vi "SingleStationGasMeter_NonNIHW.vi"() -> ()   [LabVIEW 2012]
uses:
  <vilib>/ULx/Create Channel.llb/ULx Create Channel (AI-Voltage-Basic).vi
  <vilib>/ULx/Read.llb/ULx Read (Analog DBL 1Chan 1Samp).vi
panel:
  out "ANSI Placeholder 3":dbl
  out "Start Time ANSI 3":dbl
  out "ANSI Placeholder 2":dbl
  out "Start Time ANSI 2":dbl
  out "Meter 2 Present":bool
  out "Meter 1 Present":bool
  out "Meter Type 2":string
  out "Meter Type 1":string
  out "Meter 2 Size":dbl
  out "Meter 1 Size":dbl
  out "ANSI Placeholder":dbl
  out "Start Time ANSI":dbl
  in  "Start ANSI":bool
  out "ANSI Average (BTU/hr)":dbl format="%#_5g"
  out "30 Second Average (BTU/hr)":dbl format="%#_5g"
  out "15 Second Average (BTU/hr)":dbl format="%#_5g"
  out "Reference6":dbl
  out "Reference5":dbl
  out "Reference4":dbl
  out "Reference3":dbl
  out "Reference2":dbl
  out "Reference1":dbl
  out "Time":dbl
  out "Num Record":dbl
  in  "HeatingValueLP":dbl=2450.0 min=2400.0 max=2600.0 step=5.0
  out "Output 6":dbl min=0.0 max=5.0 step=0.01
  out "Output 5":dbl min=0.0 max=5.0 step=0.01
  out "Output 4":dbl min=0.0 max=5.0 step=0.01
  out "Output 3":dbl min=0.0 max=5.0 step=0.01
  out "Output 2":dbl min=0.0 max=5.0 step=0.01
  out "Output 1":dbl min=0.0 max=5.0 step=0.01
  out "Signal":bool
  in  "Record":bool
  out "File Path":path
  out "CF/HR":dbl format="%#_2g"
  out "HV":dbl
  in  "HeatingValueNG":dbl=990.0 min=990.0 max=1150.0 step=1.0
  out "Meter ID":dbl
  out "Gas":string
  out "DisplayChart":cluster{"Flow Rate":dbl}(graph)
  out "Flow Rate":dbl format="%#_5g"
  # "Heating Value"
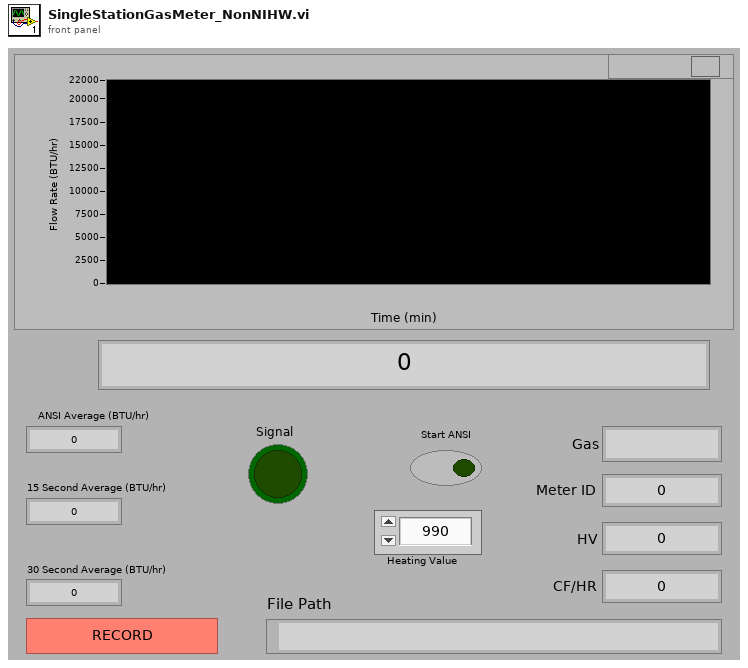
[diagram p1: front panel]
types:
  T1 = enum16{"open", "replace", "create", "open or create", "replace or create", "replace or create with confirmation"}
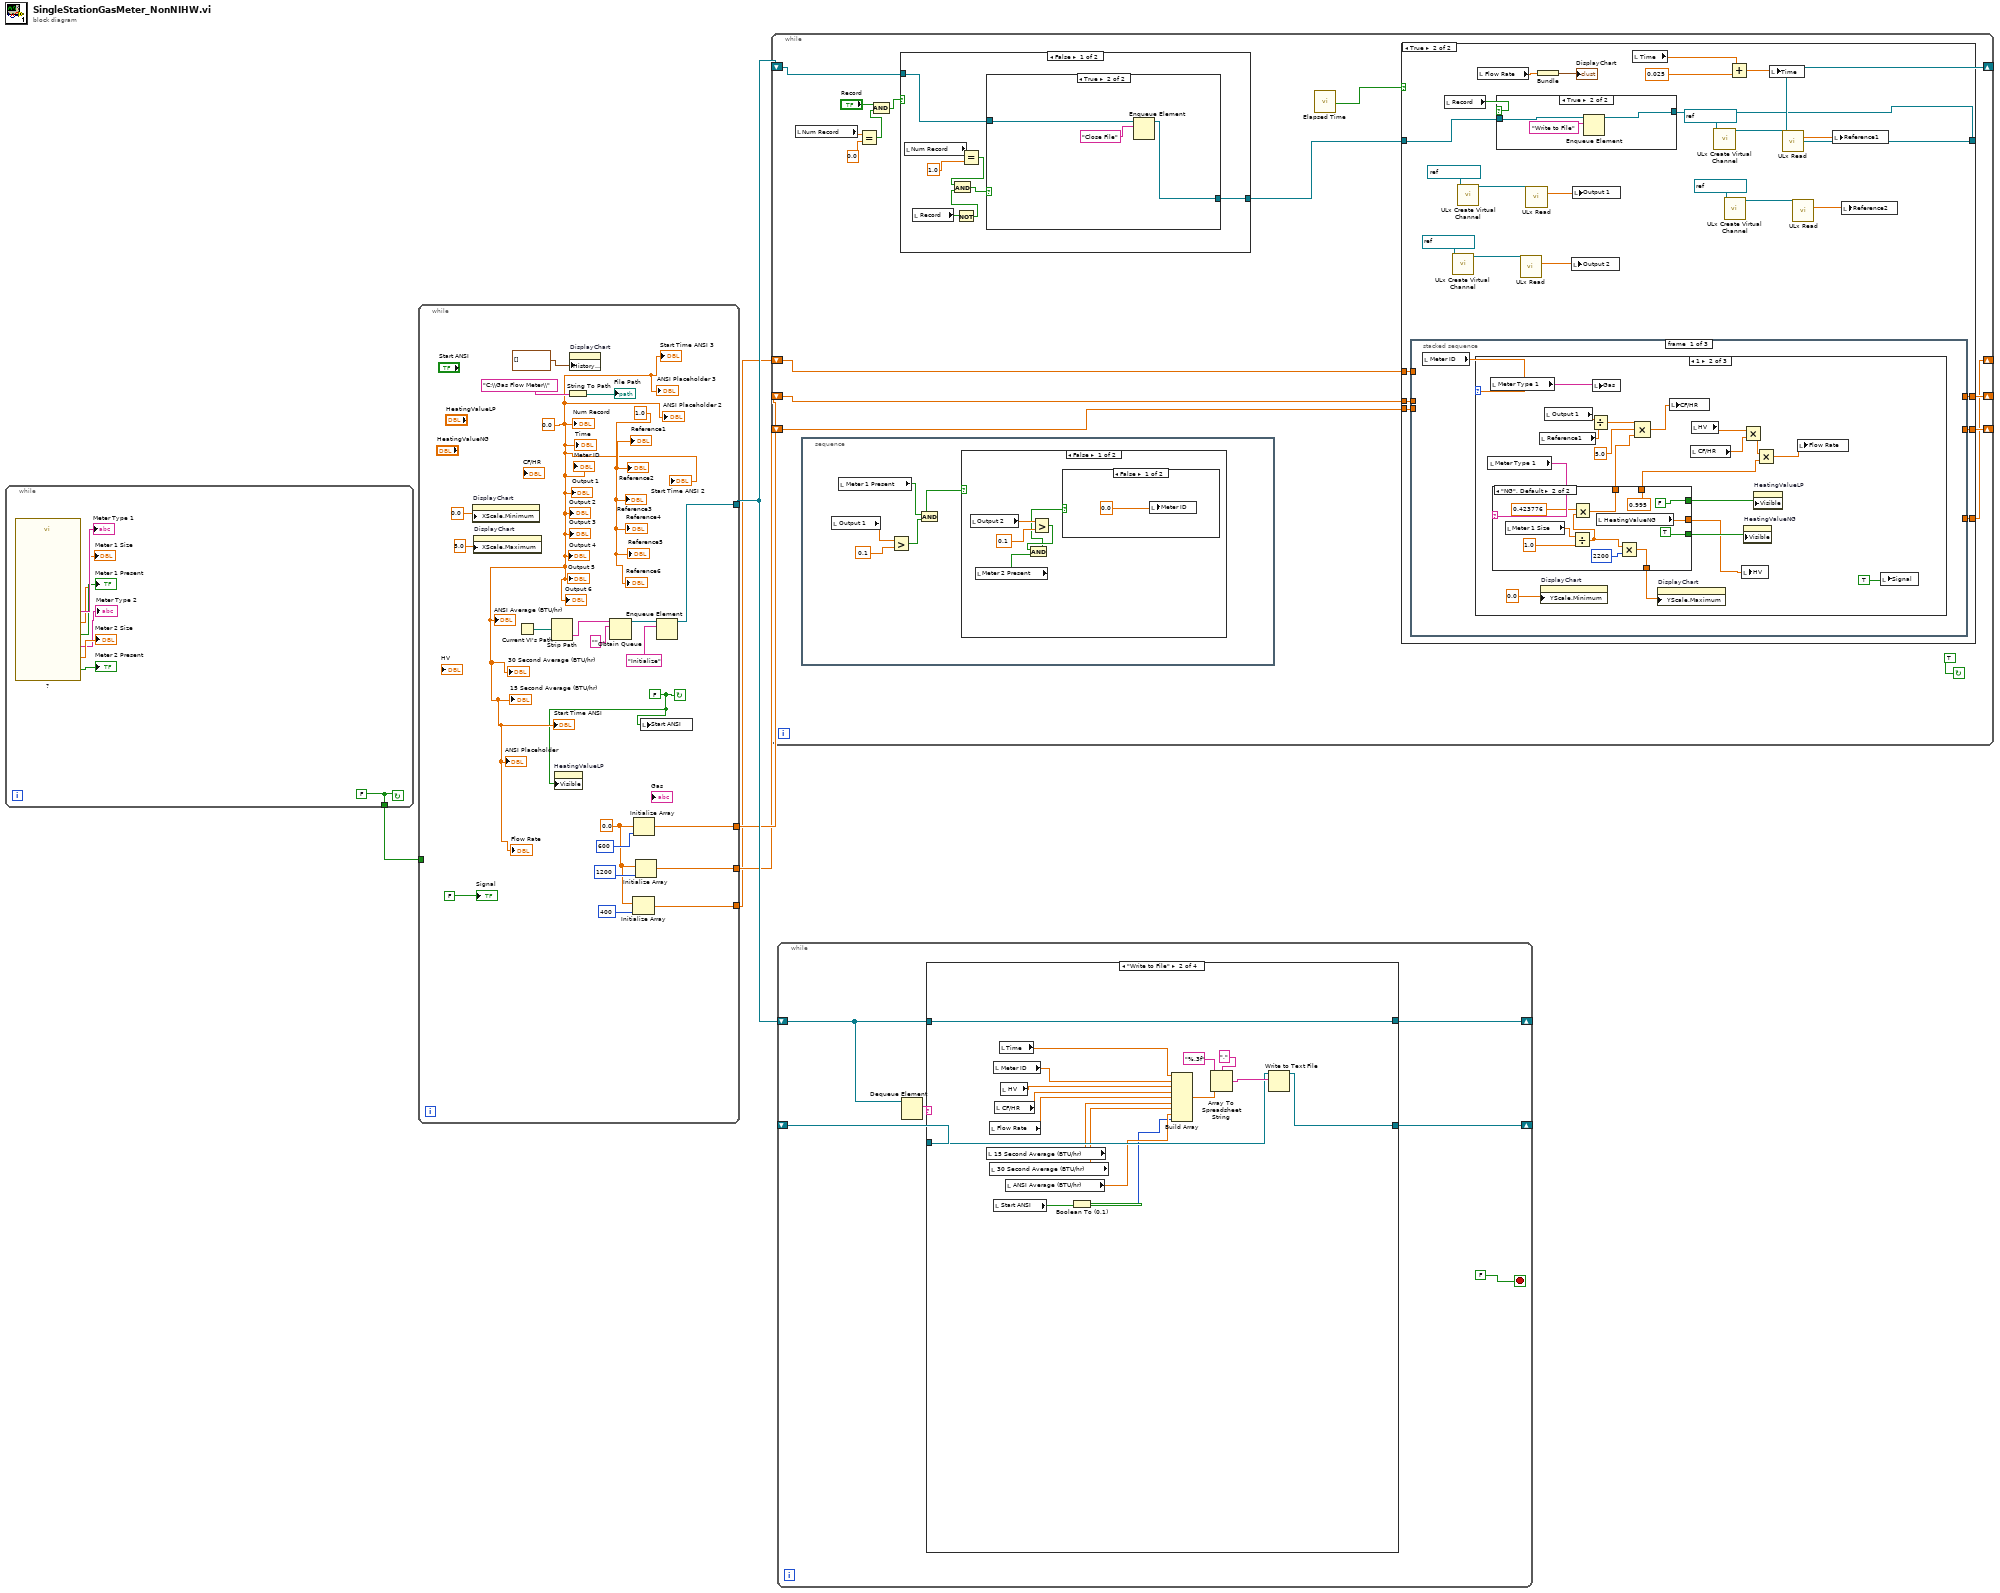
[diagram p0: block diagram]
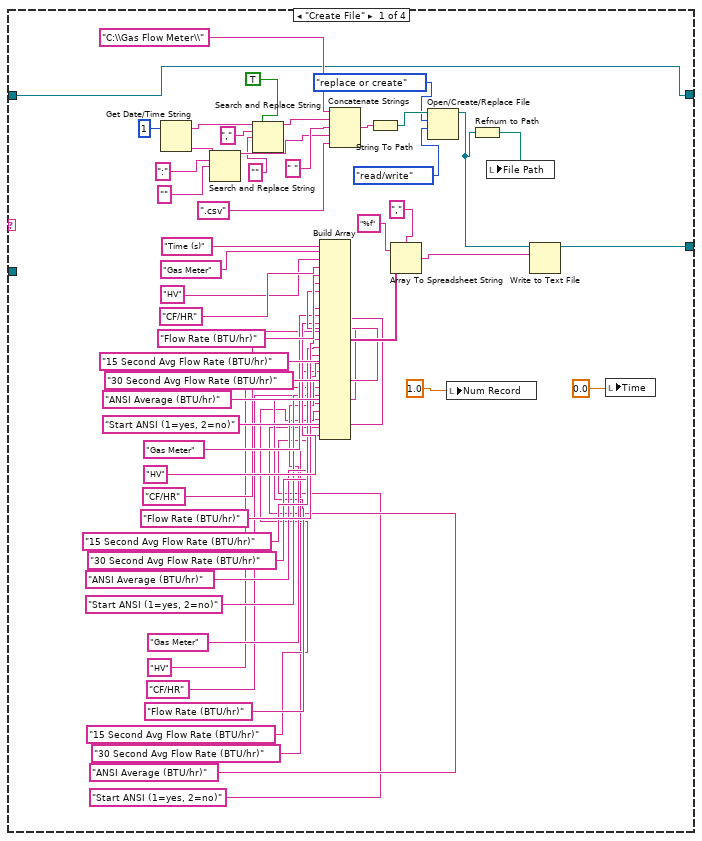
[diagram p2: hidden frame]
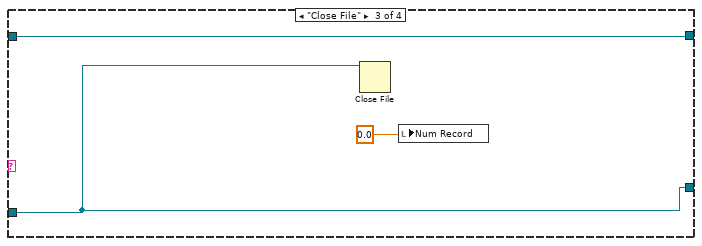
[diagram p3: hidden frame]
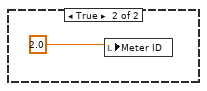
[diagram p5: hidden frame]
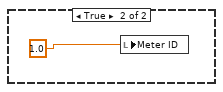
[diagram p6: hidden frame]
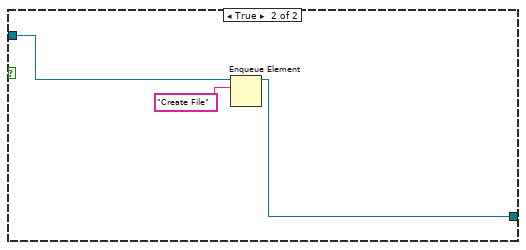
[diagram p8: hidden frame]
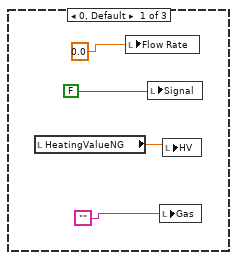
[diagram p10: hidden frame]
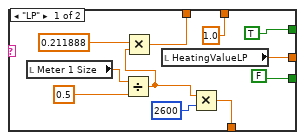
[diagram p11: hidden frame]
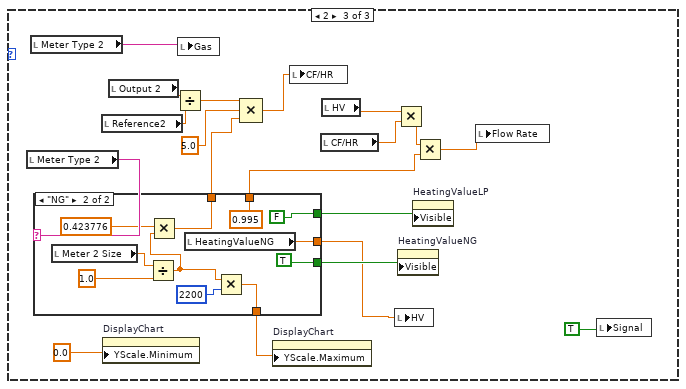
[diagram p12: hidden frame]
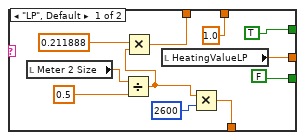
[diagram p13: hidden frame]
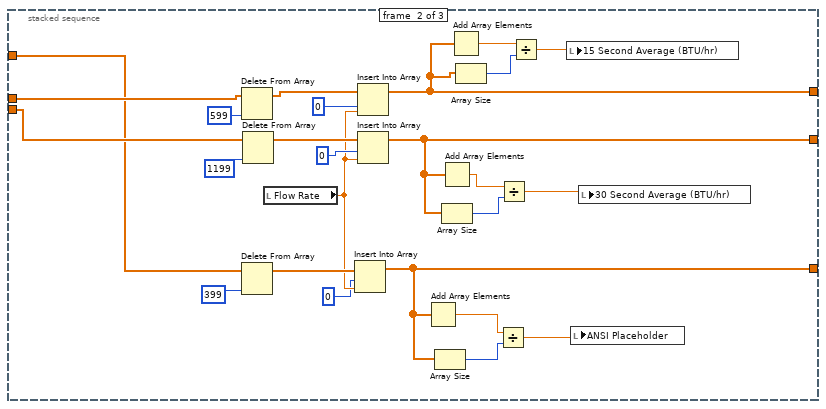
[diagram p14: hidden frame]
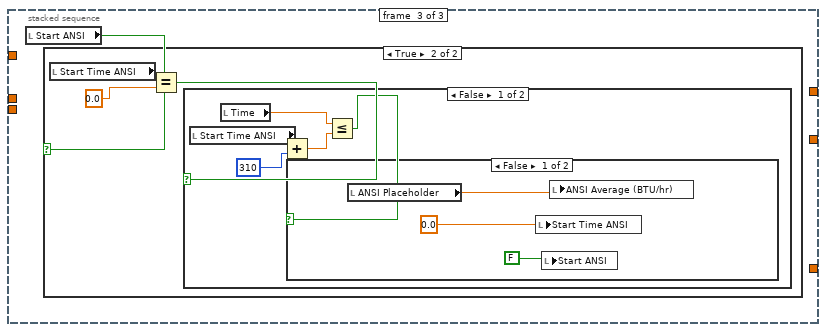
[diagram p15: hidden frame]
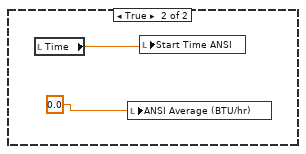
[diagram p18: hidden frame]
diagram:
  n1 = while {
    tunnel: [w11] -> w1
    stop <- w11 continue-if-true
    w11 = FALSE
    n2 = call "?"() -> ("Meter 2 Present?"=→"Meter 2 Present":bool, "Meter Size 2 (SLPM)"=→"Meter 2 Size":dbl, "Meter Type 2 (LP/NG)"=→"Meter Type 2":string, "Meter 1 Present?"=→"Meter 1 Present":bool, "Meter Size 1 (SLPM)"=→"Meter 1 Size":dbl, "Meter Type 1 (LP/NG)"=→"Meter Type 1":string)  [unwired: 12 in, 2 out]
  }
  n3 = while {
    tunnel: [w27] -> w5
    tunnel: [w23] -> w4
    tunnel: [w22] -> w3
    tunnel: [w19] -> w2
    tunnel: w1 -> [_]
    stop <- w13 continue-if-true
    w21 = 0.0
    w26 = 1.0
    w17 = 0.0
    w13 = FALSE
    n4 = property on="DisplayChart" class="WFChart (strict)"("XScale.Minimum"=0.0) -> ()  [unwired: 2 in, 2 out]
    n5 = property on="DisplayChart" class="WFChart (strict)"("XScale.Maximum"=5.0) -> ()  [unwired: 2 in, 2 out]
    n6 = Current VI's Path() -> (path=w32:path)
    n7 = Strip Path(path=w32) -> (name=w30:string)  [unwired: 1 out]
    n8 = property on="HeatingValueLP" class="DigNum (strict)"("Visible"=w13) -> ()  [unwired: 2 in, 2 out]
    n9 = String To Path(string="C:\\Gas Flow Meter\\") -> (path=→"File Path":path)
    n10 = property on="DisplayChart" class="WFChart (strict)"("History Data"=cluster{"[0]":dbl}[] []) -> ()  [unwired: 2 in, 2 out]
    n11 = Obtain Queue(name (unnamed)=w30, element data type="") -> (queue out=w28:refnum<queue>)  [unwired: 3 in, 2 out]
    n12 = Initialize Array(w21, 400) -> (w19:dbl[])
    n13 = Initialize Array(w21, 600) -> (w23:dbl[])
    n14 = Initialize Array(w21, 1200) -> (w22:dbl[])
    n15 = local write "Start ANSI"(w13) -> ()
    n16 = Enqueue Element(queue=w28, element="Initialize") -> (queue out=w27:refnum<queue>)  [unwired: 2 in, 2 out]
    "Num Record" <- w17
    "Time" <- w17
    "Meter ID" <- w17
    "Output 1" <- w17
    "Output 2" <- w17
    "Output 3" <- w17
    "Output 4" <- w17
    "Output 5" <- w17
    "Output 6" <- w17
    "Reference1" <- w26
    "Reference2" <- w26
    "Reference3" <- w26
    "Reference4" <- w26
    "Reference5" <- w26
    "Reference6" <- w26
    "30 Second Average (BTU/hr)" <- w17
    "15 Second Average (BTU/hr)" <- w17
    "ANSI Average (BTU/hr)" <- w17
    "Start Time ANSI" <- w17
    "ANSI Placeholder" <- w17
    "Flow Rate" <- w17
    "Signal" <- FALSE
    "Start Time ANSI 3" <- w17
    "ANSI Placeholder 3" <- w17
    "ANSI Placeholder 2" <- w17
    "Start Time ANSI 2" <- w17
  }
  n17 = while {
    shift-right: [w48] -> _
    shift-left: w5 -> [w41]
    shift-right: [w47] -> _
    shift-left: w4 -> [w45]
    shift-right: [w46] -> _
    shift-left: w3 -> [w44]
    shift-right: [w43] -> _
    shift-left: w2 -> [w42]
    stop <- TRUE continue-if-true
    n18 = local read "Num Record"() -> (w37:dbl)
    n19 = stacked-sequence {
      frame #0 {
        n20 = local read "Output 1"() -> (w55:dbl)
        n21 = local read "Meter 1 Present"() -> (w52:bool)
        n22 = Greater?(x=w55, y=0.1) -> (0:w53:bool)
        n23 = And(x=w52, y=w53) -> (x .and. y?=w51:bool)
        n24 = case shown="False" w51 {
          frame False {
            n25 = local read "Output 2"() -> (w59:dbl)
            n26 = local read "Meter 2 Present"() -> (w58:bool)
            n27 = Greater?(x=w59, y=0.1) -> (0:w57:bool)
            n28 = And(x=w57, y=w58) -> (x .and. y?=w56:bool)
            n29 = case shown="False" w56 {
              frame False {
                n30 = local write "Meter ID"(0.0) -> ()
              }
              frame True {
                n31 = local write "Meter ID"(2.0) -> ()
              }
            }
          }
          frame True {
            n32 = local write "Meter ID"(1.0) -> ()
          }
        }
      }
    }
    n33 = Equal?(x=w37, y=0.0) -> (x = y?=w36:bool)
    n34 = And(x="Record", y=w36) -> (x .and. y?=w35:bool)
    n35 = case shown="False" w35 {
      tunnel: w41 -> [w69 w77]
      tunnel: [w68 w76] -> w40
      frame False {
        n36 = local read "Num Record"() -> (w71:dbl)
        n37 = local read "Record"() -> (w65:bool)
        n38 = Not(x=w65) -> (.not. x?=w64:bool)
        n39 = Equal?(x=w71, y=1.0) -> (x = y?=w67:bool)
        n40 = And(x=w67, y=w64) -> (x .and. y?=w66:bool)
        n41 = case shown="True" w66 {
          tunnel: w69 -> [w72 w74]
          tunnel: [w72 w73] -> w68
          frame False {
          }
          frame True {
            n42 = Enqueue Element(queue=w74, element="Close File") -> (queue out=w73:refnum<queue>)  [unwired: 2 in, 2 out]
          }
        }
      }
      frame True {
        n43 = Enqueue Element(queue=w77, element="Create File") -> (queue out=w76:refnum<queue>)  [unwired: 2 in, 2 out]
      }
    }
    n44 = call "Elapsed Time"() -> ("Time has Elapsed"=w49:bool)  [unwired: 12 in, 7 out]
    n45 = case shown="True" w49 {
      tunnel: w40 -> [w82 w103]
      tunnel: [w82 w102] -> w48
      tunnel: w45 -> [w81 w101]
      tunnel: w44 -> [w80 w100]
      tunnel: [w81 w99] -> w47
      tunnel: [w80 w98] -> w46
      tunnel: w42 -> [w79 w97]
      tunnel: [w79 w96] -> w43
      frame False {
      }
      frame True {
        n46 = stacked-sequence {
          tunnel: w101 -> [_ w220 _]
          tunnel: w100 -> [_ w219 _]
          tunnel: [_ w214 _] -> w99
          tunnel: [_ w210 _] -> w98
          tunnel: w97 -> [_ w204 _]
          tunnel: [_ w201 _] -> w96
          frame #0 {
            n47 = local read "Meter ID"() -> (w109:dbl)
            n48 = case shown="1" w109 {
              frame 0, Default {
                n49 = local read "HeatingValueNG"() -> (w113:dbl)
                n50 = local write "Flow Rate"(0.0) -> ()
                n51 = local write "Signal"(FALSE) -> ()
                n52 = local write "Gas"("") -> ()
                n53 = local write "HV"(w113) -> ()
              }
              frame 1 {
                n54 = local read "Meter Type 1"() -> (w122:string)
                n55 = local read "Meter Type 1"() -> (w116:string)
                n56 = case shown="\"NG\", Default" w122 {
                  tunnel: [w140 w151] -> w121
                  tunnel: [TRUE FALSE] -> w120
                  tunnel: [FALSE TRUE] -> w119
                  tunnel: [1.0 0.995] -> w118
                  tunnel: [w134 w145] -> w117
                  tunnel: [w133 w144] -> w115
                  frame "LP" {
                    n57 = local read "Meter 1 Size"() -> (w142:dbl)
                    n58 = Divide(x=w142, y=0.5) -> (x/y=w135:dbl)
                    n59 = Multiply(x=0.211888, y=w135) -> (x*y=w140:dbl)
                    n60 = local read "HeatingValueLP"() -> (w133:dbl)
                    n61 = Multiply(x=w135, y=2600) -> (x*y=w134:dbl)
                  }
                  frame "NG", Default {
                    n62 = local read "Meter 1 Size"() -> (w153:dbl)
                    n63 = Divide(x=w153, y=1.0) -> (x/y=w146:dbl)
                    n64 = Multiply(x=0.423776, y=w146) -> (x*y=w151:dbl)
                    n65 = local read "HeatingValueNG"() -> (w144:dbl)
                    n66 = Multiply(x=w146, y=2200) -> (x*y=w145:dbl)
                  }
                }
                n67 = local read "Reference1"() -> (w126:dbl)
                n68 = property on="DisplayChart" class="WFChart (strict)"("YScale.Minimum"=0.0) -> ()  [unwired: 2 in, 2 out]
                n69 = local read "Output 1"() -> (w127:dbl)
                n70 = Divide(x=w127, y=w126) -> (x/y=w124:dbl)
                n71 = local write "Gas"(w116) -> ()
                n72 = Compound Arithmetic op=MULTIPLY(w124, 5.0, w121) -> (w114:dbl)
                n73 = property on="DisplayChart" class="WFChart (strict)"("YScale.Maximum"=w117) -> ()  [unwired: 2 in, 2 out]
                n74 = local write "CF/HR"(w114) -> ()
                n75 = local read "CF/HR"() -> (w129:dbl)
                n76 = local read "HV"() -> (w128:dbl)
                n77 = local write "HV"(w115) -> ()
                n78 = Multiply(x=w128, y=w129) -> (x*y=w130:dbl)
                n79 = property on="HeatingValueNG" class="DigNum (strict)"("Visible"=w119) -> ()  [unwired: 2 in, 2 out]
                n80 = property on="HeatingValueLP" class="DigNum (strict)"("Visible"=w120) -> ()  [unwired: 2 in, 2 out]
                n81 = Multiply(x=w130, y=w118) -> (x*y=w131:dbl)
                n82 = local write "Flow Rate"(w131) -> ()
                n83 = local write "Signal"(TRUE) -> ()
              }
              frame 2 {
                n84 = local read "Meter Type 2"() -> (w163:string)
                n85 = local read "Meter Type 2"() -> (w157:string)
                n86 = case shown="\"NG\"" w163 {
                  tunnel: [w181 w192] -> w162
                  tunnel: [TRUE FALSE] -> w161
                  tunnel: [FALSE TRUE] -> w160
                  tunnel: [1.0 0.995] -> w159
                  tunnel: [w175 w186] -> w158
                  tunnel: [w174 w185] -> w156
                  frame "LP", Default {
                    n87 = local read "Meter 2 Size"() -> (w183:dbl)
                    n88 = Divide(x=w183, y=0.5) -> (x/y=w176:dbl)
                    n89 = Multiply(x=0.211888, y=w176) -> (x*y=w181:dbl)
                    n90 = local read "HeatingValueLP"() -> (w174:dbl)
                    n91 = Multiply(x=w176, y=2600) -> (x*y=w175:dbl)
                  }
                  frame "NG" {
                    n92 = local read "Meter 2 Size"() -> (w194:dbl)
                    n93 = Divide(x=w194, y=1.0) -> (x/y=w187:dbl)
                    n94 = Multiply(x=0.423776, y=w187) -> (x*y=w192:dbl)
                    n95 = local read "HeatingValueNG"() -> (w185:dbl)
                    n96 = Multiply(x=w187, y=2200) -> (x*y=w186:dbl)
                  }
                }
                n97 = local read "Reference2"() -> (w167:dbl)
                n98 = property on="DisplayChart" class="WFChart (strict)"("YScale.Minimum"=0.0) -> ()  [unwired: 2 in, 2 out]
                n99 = local read "Output 2"() -> (w168:dbl)
                n100 = Divide(x=w168, y=w167) -> (x/y=w165:dbl)
                n101 = local write "Gas"(w157) -> ()
                n102 = Compound Arithmetic op=MULTIPLY(w165, 5.0, w162) -> (w155:dbl)
                n103 = property on="DisplayChart" class="WFChart (strict)"("YScale.Maximum"=w158) -> ()  [unwired: 2 in, 2 out]
                n104 = local write "CF/HR"(w155) -> ()
                n105 = local read "CF/HR"() -> (w170:dbl)
                n106 = local read "HV"() -> (w169:dbl)
                n107 = local write "HV"(w156) -> ()
                n108 = Multiply(x=w169, y=w170) -> (x*y=w171:dbl)
                n109 = property on="HeatingValueNG" class="DigNum (strict)"("Visible"=w160) -> ()  [unwired: 2 in, 2 out]
                n110 = property on="HeatingValueLP" class="DigNum (strict)"("Visible"=w161) -> ()  [unwired: 2 in, 2 out]
                n111 = Multiply(x=w171, y=w159) -> (x*y=w172:dbl)
                n112 = local write "Flow Rate"(w172) -> ()
                n113 = local write "Signal"(TRUE) -> ()
              }
            }
          }
          frame #1 {
            n114 = Delete From Array(array=w220, index=599) -> (array with subset deleted=w215:dbl[])  [unwired: 1 in, 1 out]
            n115 = Delete From Array(array=w204, index=399) -> (array with subset deleted=w202:dbl[])  [unwired: 1 in, 1 out]
            n116 = Delete From Array(array=w219, index=1199) -> (array with subset deleted=w216:dbl[])  [unwired: 1 in, 1 out]
            n117 = local read "Flow Rate"() -> (w197:dbl)
            n118 = Insert Into Array(array=w202, index=0, new element=w197) -> (w201:dbl[])
            n119 = Insert Into Array(array=w215, index=0, new element=w197) -> (w214:dbl[])
            n120 = Insert Into Array(array=w216, index=0, new element=w197) -> (w210:dbl[])
            n121 = Add Array Elements(numeric array=w201) -> (sum=w200:dbl)
            n122 = Array Size(array=w201) -> (size(s)=w199:i32)
            n123 = Add Array Elements(numeric array=w210) -> (sum=w209:dbl)
            n124 = Array Size(array=w210) -> (size(s)=w208:i32)
            n125 = Add Array Elements(numeric array=w214) -> (sum=w212:dbl)
            n126 = Array Size(array=w214) -> (size(s)=w213:i32)
            n127 = Divide(x=w200, y=w199) -> (x/y=w198:dbl)
            n128 = Divide(x=w209, y=w208) -> (x/y=w207:dbl)
            n129 = Divide(x=w212, y=w213) -> (x/y=w211:dbl)
            n130 = local write "15 Second Average (BTU/hr)"(w211) -> ()
            n131 = local write "ANSI Placeholder"(w198) -> ()
            n132 = local write "30 Second Average (BTU/hr)"(w207) -> ()
          }
          frame #2 {
            n133 = local read "Start ANSI"() -> (w221:bool)
            n134 = case shown="True" w221 {
              frame False {
              }
              frame True {
                n135 = local read "Start Time ANSI"() -> (w223:dbl)
                n136 = Equal?(x=w223, y=0.0) -> (x = y?=w222:bool)
                n137 = case shown="False" w222 {
                  frame False {
                    n138 = local read "Start Time ANSI"() -> (w229:dbl)
                    n139 = local read "Time"() -> (w226:dbl)
                    n140 = Add(x=w229, y=310) -> (x+y=w227:dbl)
                    n141 = Less Or Equal?(x=w226, y=w227) -> (x <= y?=w225:bool)
                    n142 = case shown="False" w225 {
                      frame False {
                        n143 = local read "ANSI Placeholder"() -> (w231:dbl)
                        n144 = local write "Start Time ANSI"(0.0) -> ()
                        n145 = local write "Start ANSI"(FALSE) -> ()
                        n146 = local write "ANSI Average (BTU/hr)"(w231) -> ()
                      }
                      frame True {
                      }
                    }
                  }
                  frame True {
                    n147 = local read "Time"() -> (w234:dbl)
                    n148 = local write "ANSI Average (BTU/hr)"(0.0) -> ()
                    n149 = local write "Start Time ANSI"(w234) -> ()
                  }
                }
              }
            }
          }
        }
        n150 = local read "Record"() -> (w106:bool)
        n151 = call-poly <vilib>:"ULx Create Virtual Channel.vi"("physical channels"=refnum<k21> "Dev0/Ai3") -> ("task out"=w87:refnum<k24>)  [unwired: 13 in, 1 out]
        n152 = call-poly <vilib>:"ULx Create Virtual Channel.vi"("physical channels"=refnum<k21> "Dev0/Ai2") -> ("task out"=w89:refnum<k24>)  [unwired: 13 in, 1 out]
        n153 = local read "Flow Rate"() -> (w108:dbl)
        n154 = case shown="True" w106 {
          tunnel: w103 -> [w235 w237]
          tunnel: [w235 w236] -> w102
          frame False {
          }
          frame True {
            n155 = Enqueue Element(queue=w237, element="Write to File") -> (queue out=w236:refnum<queue>)  [unwired: 2 in, 2 out]
          }
        }
        n156 = call-poly <vilib>:"ULx Read.vi"("task in"=w87) -> ("data"=w85:dbl)  [unwired: 12 in, 2 out]
        n157 = call-poly <vilib>:"ULx Read.vi"("task in"=w89) -> ("data"=w86:dbl)  [unwired: 12 in, 2 out]
        n158 = Bundle("Flow Rate"=w108) -> (→"DisplayChart":cluster{"Flow Rate":dbl})  [unwired: 1 in]
        n159 = local write "Output 2"(w85) -> ()
        n160 = local write "Output 1"(w86) -> ()
        n161 = local read "Time"() -> (w105:dbl)
        n162 = call-poly <vilib>:"ULx Create Virtual Channel.vi"("physical channels"=refnum<k21> "Dev0/Ai0") -> ("task out"=w94:refnum<k24>)  [unwired: 13 in, 1 out]
        n163 = call-poly <vilib>:"ULx Create Virtual Channel.vi"("physical channels"=refnum<k21> "Dev0/Ai1") -> ("task out"=w91:refnum<k24>)  [unwired: 13 in, 1 out]
        n164 = Add(x=w105, y=0.025) -> (x+y=w104:dbl)
        n165 = local write "Time"(w104) -> ()
        n166 = call-poly <vilib>:"ULx Read.vi"("task in"=w94) -> ("data"=w93:dbl)  [unwired: 12 in, 2 out]
        n167 = call-poly <vilib>:"ULx Read.vi"("task in"=w91) -> ("data"=w84:dbl)  [unwired: 12 in, 2 out]
        n168 = local write "Reference1"(w93) -> ()
        n169 = local write "Reference2"(w84) -> ()
      }
    }
  }
  n170 = while {
    shift-right: [w242] -> _
    shift-left: w5 -> [w239]
    shift-right: [w241] -> _
    shift-left: _ -> [w240]
    stop <- FALSE stop-if-true
    n171 = Dequeue Element(queue=w239) -> (element=w243:string)  [unwired: 2 in, 3 out]
    n172 = case shown="\"Write to File\"" w243 {
      tunnel: [w266 w304 w315 w318] -> w242
      tunnel: w239 -> [w266 w304 w315 w318]
      tunnel: [w265 w302 w314 w317] -> w241
      tunnel: w240 -> [_ w303 w314 w317]
      frame "Create File" {
        n173 = Get Date/Time String(date format (0)=1) -> (date string=w271:string, time string=w268:string)  [unwired: 2 in]
        n174 = Search and Replace String(input string=w268, search string=":", replace string="") -> (result string=w277:string)  [unwired: 5 in, 3 out]
        n175 = Search and Replace String(replace all?=TRUE, input string=w271, search string=",", replace string="") -> (result string=w278:string)  [unwired: 4 in, 3 out]
        n176 = Build Array("Time (s)", "Gas Meter", "HV", "CF/HR", "Flow Rate (BTU/hr)", "15 Second Avg Flow Rate (BTU/hr)", "30 Second Avg Flow Rate (BTU/hr)", "ANSI Average (BTU/hr)", "Start ANSI (1=yes, 2=no)", "Gas Meter", "HV", "CF/HR", "Flow Rate (BTU/hr)", "15 Second Avg Flow Rate (BTU/hr)", "30 Second Avg Flow Rate (BTU/hr)", "ANSI Average (BTU/hr)", "Start ANSI (1=yes, 2=no)", "Gas Meter", "HV", "CF/HR", "Flow Rate (BTU/hr)", "15 Second Avg Flow Rate (BTU/hr)", "30 Second Avg Flow Rate (BTU/hr)", "ANSI Average (BTU/hr)", "Start ANSI (1=yes, 2=no)") -> (w288:string[])
        n177 = Concatenate Strings("C:\\Gas Flow Meter\\", w278, " ", w277, ".csv") -> (w274:string)
        n178 = String To Path(string=w274) -> (path=w294:path)
        n179 = Array To Spreadsheet String(delimiter (Tab)=",", array=w288, 3:"%f" ("format string")) -> (spreadsheet string=w289:string)
        n180 = Open/Create/Replace File(file path (use dialog)=w294, operation (0:open)=T1."replace or create", access (0:read/write)=enum16{"read/write", "read-only", "write-only"}."read/write") -> (refnum out=w296:refnum<file>)  [unwired: 3 in, 2 out]
        n181 = local write "Num Record"(1.0) -> ()
        n182 = Refnum to Path(1:w296) -> (0:w295:path)
        n183 = local write "File Path"(w295) -> ()
        n184 = Write to Text File(file (use dialog)=w296, text=w289) -> (refnum out=w265:refnum<file>)  [unwired: 2 in, 2 out]
        n185 = local write "Time"(0.0) -> ()
      }
      frame "Write to File" {
        n186 = local read "15 Second Average (BTU/hr)"() -> (w300:dbl)
        n187 = local read "Flow Rate"() -> (w307:dbl)
        n188 = local read "30 Second Average (BTU/hr)"() -> (w301:dbl)
        n189 = local read "Meter ID"() -> (w310:dbl)
        n190 = local read "Start ANSI"() -> (w298:bool)
        n191 = local read "CF/HR"() -> (w308:dbl)
        n192 = local read "Time"() -> (w311:dbl)
        n193 = local read "HV"() -> (w309:dbl)
        n194 = local read "ANSI Average (BTU/hr)"() -> (w299:dbl)
        n195 = Boolean To (0,1)(Boolean=w298) -> (0, 1=w297:i16)
        n196 = Build Array(w311, w310, w309, w308, w307, w300, w301, w299, w297) -> (w306:dbl[])
        n197 = Array To Spreadsheet String(delimiter (Tab)=",", array=w306, 3:"%.3f" ("format string")) -> (spreadsheet string=w305:string)
        n198 = Write to Text File(file (use dialog)=w303, text=w305) -> (refnum out=w302:refnum<file>)  [unwired: 2 in, 2 out]
      }
      frame "Close File" {
        n199 = Close File(refnum=w314) -> ()  [unwired: 1 in, 2 out]
        n200 = local write "Num Record"(0.0) -> ()
      }
      frame "Initialize", Default {
      }
    }
  }
